vi "Untitled 7 (SubVI).vi"(8 "error in (no error)":errorcluster, 10 "Angle (degrees)":sgl format="%.2f", 11 "Refnum in":T3) -> (0 "error out":errorcluster, 1 "Number of Matches (Geometric Matching 1)":i32, 2 "Image Out":T2, 3 "Refnum out":T3, 4 "Calibrated Matches (Geometric Matching 1)":T1[](array[typedef]) {"Correlation Score" format="%.2f"; "Target Template Curve Score" format="%.2f"; "Template Target Curve Score" format="%.2f"; "Bounding Box"."y" format="%.2f"; "Bounding Box"."x" format="%.2f"; "Position"."y" format="%.2f"; "Position"."x" format="%.2f"; "Score" format="%.2f"; "Scale" format="%.2f"; "Angle" format="%.2f"; "Occlusion %" format="%.2f"})   [LabVIEW 2017]
uses:
  <vilib>/userdefined/High Color/IMAQdx.ctl
  <vilib>/vision/Image Controls.llb/IMAQ Image.ctl
  <vilib>/vision/Pattern Matching.llb/IMAQ GM Match Report.ctl
  <vilib>/vision/NI_Vision_Development_Module.lvlib
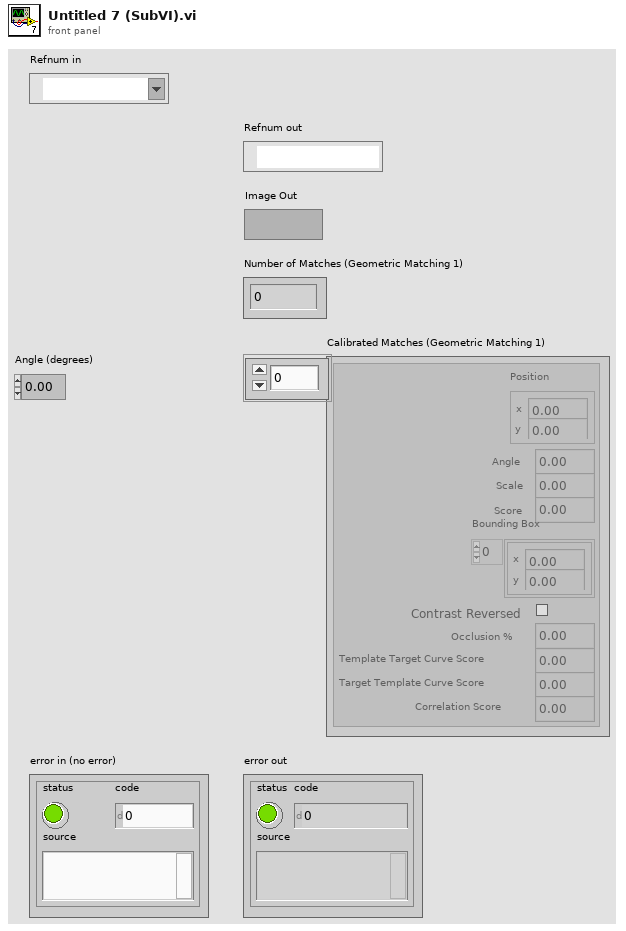
[diagram p1: front panel]
types:
  T1 = typedef "IMAQ GM Match Report.ctl" = cluster{"Position":cluster{"x":sgl, "y":sgl}, "Angle":sgl, "Scale":sgl, "Score":sgl, "Bounding Box":cluster{"x":sgl, "y":sgl}[], "Contrast Reversed":bool, "Occlusion %":sgl, "Template Target Curve Score":sgl, "Target Template Curve Score":sgl, "Correlation Score":sgl}
  T2 = typedef "IMAQ Image.ctl" = refnum<image>
  T3 = typedef "IMAQdx.ctl" = refnum<k21>
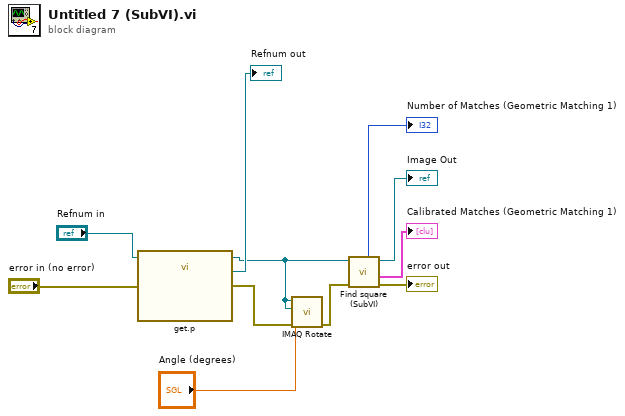
[diagram p0: block diagram]
diagram:
  n1 = call "get.p.vi"("Session in"="Refnum in", "error in"="error in (no error)") -> ("Image Out"=w1:T2, "Session Out"=→"Refnum out":T3, "error out"=w3:errorcluster)  [unwired: 23 in]
  n2 = call "IMAQ Rotate"("error in (no error)"=w3, "Angle (degrees)"="Angle (degrees)", "Image Dst"=w1, "Image Src"=w1) -> ("error out"=w2:errorcluster)  [unwired: 6 in, 1 out]
  n3 = call "Find square (SubVI).vi"("error in (no error)"=w2, "Refnum in"=w1) -> ("error out"=→"error out":errorcluster, "Calibrated Matches (Geometric Matching 1)"=→"Calibrated Matches (Geometric Matching 1)":T1[], "Refnum out"=→"Image Out":T2, "Number of Matches (Geometric Matching 1)"=→"Number of Matches (Geometric Matching 1)":i32)  [unwired: 5 in, 1 out]
